vi "Teleop.vi"(10 "Match Info":T1={"Autonomous Elapsed Seconds"=0.0, "TeleOp Elapsed Seconds"=0.0, "Disabled Elapsed Seconds"=0.0, "Visited Autonomous"=FALSE, "Visited TeleOp"=FALSE, "Visited Disabled"=FALSE, "Autonomous Settings"={"Autonomous Style"=enum."Independent", "VI Refnum"=refnum}}, 11 "Call Context":T2) -> ()   [LabVIEW 2011]
doc: "This VI is called for each TeleOp packet received from the DS where the robot is not disabled. It is often used to read from the joysticks and update I/O or to update setpoints for timed control loops. It should complete and return within 20 milliseconds or it may miss DS packets."
uses:
  <vilib>/Rock Robotics/WPI/DriverStation/WPI_DriverStationDerivedRobotMode.ctl
  <vilib>/Rock Robotics/WPI/DriverStation/WPI_DriverStationMatch Info.ctl
  <vilib>/Rock Robotics/WPI/Relay/WPI_RelayValue.ctl
  Robot Global Data.vi
panel:
  out "Shift Control":dbl=2.0 format="%.2f"
  in  "Left High":dbl=0.2
  in  "Right High":dbl=0.8
  in  "Left Mid":dbl=0.25
  in  "Right Mid":dbl=0.7
  in  "Shift Input 2":dbl
  in  "Left Low":dbl=0.8
  in  "Right Low":dbl=0.4
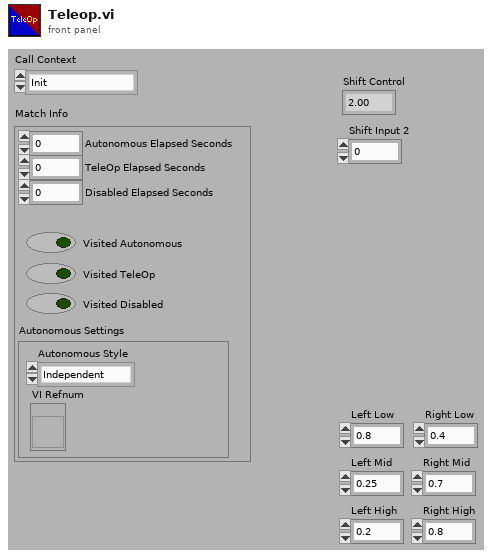
[diagram p1: front panel]
types:
  T1 = typedef "WPI_DriverStationMatch Info.ctl" = cluster{"Autonomous Elapsed Seconds":dbl, "TeleOp Elapsed Seconds":dbl, "Disabled Elapsed Seconds":dbl, "Visited Autonomous":bool, "Visited TeleOp":bool, "Visited Disabled":bool, "Autonomous Settings":cluster{"Autonomous Style":enum16{"Iterative", "Independent"}, "VI Refnum":refnum<vi>}}
  T2 = typedef "WPI_DriverStationDerivedRobotMode.ctl" = enum16{"Init", "Execute", "Stop"}
  T3 = typedef "WPI_RelayValue.ctl" = enum16{"Off", "On", "Forward", "Reverse"}
  T4 = typedef "WPI_MotorControlDeviceRef.ctl" = cluster{"DeviceStatus":errorcluster, "Type":enum16{"PWM", "CAN"}, "PWM":cluster{"Digital Module":T5, "PWM Channel":T6, "DeadBand":T7}, "CAN":cluster{"Device Number":u8, "Control Mode":T8, "Semaphore":T9, "Max Vout":dbl}, "Invert":bool, "TransformRef":T10, "InvTransformRef":T10}
  T5 = typedef "FPGA_TypedefDigitalModule.ctl" = enum16{"Digital Module 1", "Digital Module 2"}
  T6 = typedef "FPGA_DIOPWMChannel.ctl" = enum8{"PWM 1", "PWM 2", "PWM 3", "PWM 4", "PWM 5", "PWM 6", "PWM 7", "PWM 8", "PWM 9", "PWM 10", "Invalid"}
  T7 = typedef "WPI_PWMDeadband.ctl" = cluster{"Name":string, "maxPositivePwm":i32, "minPositivePwm":i32, "centerPwm":i32, "maxNegativePwm":i32, "minNegativePwm":i32, "angularRange":u16}
  T8 = typedef "WPI_CANJaguar_ControlMode.ctl" = enum8{"Percent VBus", "Current", "Speed", "Position", "Voltage"}
  T9 = typedef "Semaphore RefNum" = refnum<k1>
  T10 = typedef "WPI_PWMTransform_ConPane.ctl" = refnum<vi>
  T11 = typedef "WPI_RelayDevRef.ctl" = cluster{"DevStatus":errorcluster, "Relay Channel":T12, "Digital Module":T5, "Relay Direction":T13}
  T12 = typedef "FPGA_DIORelayChannel.ctl" = enum8{"Relay 1", "Relay 2", "Relay 3", "Relay 4", "Relay 5", "Relay 6", "Relay 7", "Relay 8", "Invalid"}
  T13 = typedef "WPI_RelayDirection.ctl" = enum16{"Both directions", "Forward only", "Reverse only"}
  T14 = typedef "WPI_ServoDeviceRef.ctl" = cluster{"DeviceStatus":errorcluster, "Digital Module":T5, "PWM Channel":T6, "DeadBand":T7}
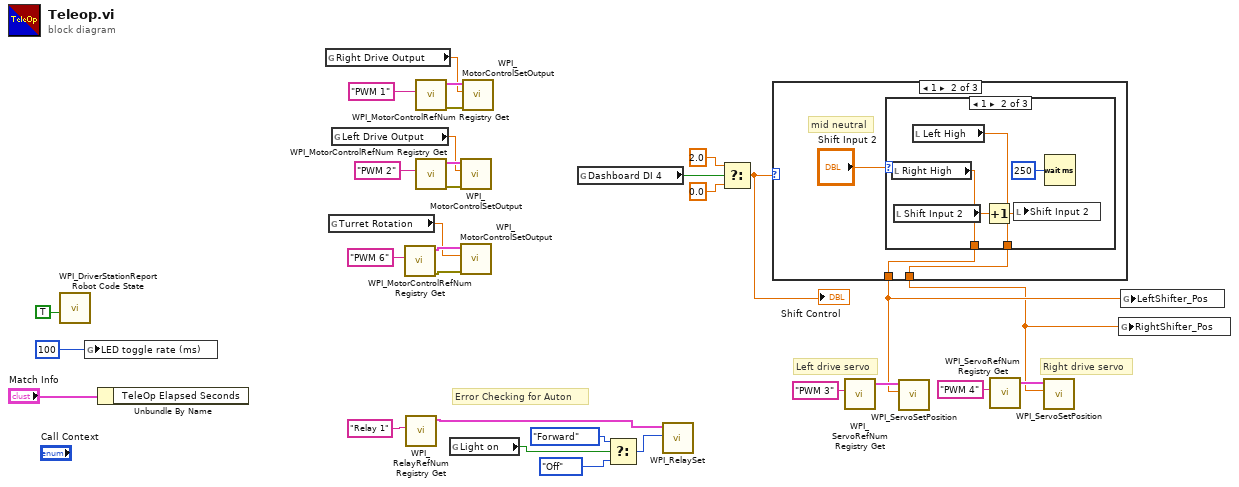
[diagram p0: block diagram]
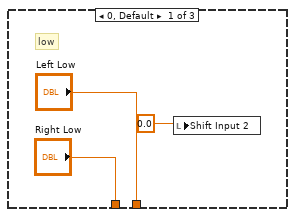
[diagram p2: hidden frame]
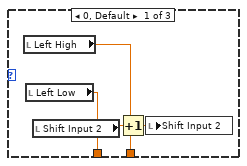
[diagram p3: hidden frame]
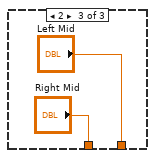
[diagram p4: hidden frame]
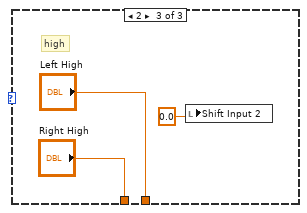
[diagram p5: hidden frame]
diagram:
  # "Error Checking for Auton"
  # "Right drive servo"
  # "Left drive servo"
  n1 = call <vilib>:"WPI_DriverStationReport Robot Code State.vi"("TeleOp"=TRUE ("Autonomous")) -> ()  [unwired: 10 in, 1 out]
  n2 = global write "Robot Global Data.vi" "LED toggle rate (ms)"(u32 100 ("LED ms toggle rate")) -> ()
  n3 = Unbundle By Name("Match Info") -> ()  [unwired: 1 out]
  n4 = global read "Robot Global Data.vi" "Right Drive Output"() -> (w7:dbl)
  n5 = global read "Robot Global Data.vi" "Turret Rotation"() -> (w9:dbl)
  n6 = global read "Robot Global Data.vi" "Left Drive Output"() -> (w8:dbl)
  n7 = call <vilib>:"WPI_MotorControlRefNum Registry Get.vi"("refnum name"="PWM 6") -> ("error out"=w12:errorcluster, "MotorControlDevRef"=w11:T4)  [unwired: 9 in]
  n8 = call <vilib>:"WPI_RelayRefNum Registry Get.vi"("refnum name"="Relay 1") -> ("RelayDevRef"=w1:T11)  [unwired: 9 in, 1 out]
  n9 = call <vilib>:"WPI_MotorControlRefNum Registry Get.vi"("refnum name"="PWM 1") -> ("error out"=w25:errorcluster, "MotorControlDevRef"=w26:T4)  [unwired: 9 in]
  n10 = call <vilib>:"WPI_MotorControlRefNum Registry Get.vi"("refnum name"="PWM 2") -> ("error out"=w23:errorcluster, "MotorControlDevRef"=w24:T4)  [unwired: 9 in]
  n11 = global read "Robot Global Data.vi" "Light on"() -> (w4:bool)
  n12 = call <vilib>:"WPI_MotorControlSetOutput.vi"("error in (no error)"=w23, "Output"=w8, "MotorControlDevRef"=w24) -> ()  [unwired: 7 in, 2 out]
  n13 = call <vilib>:"WPI_MotorControlSetOutput.vi"("error in (no error)"=w12, "Output"=w9, "MotorControlDevRef"=w11) -> ()  [unwired: 7 in, 2 out]
  n14 = call <vilib>:"WPI_MotorControlSetOutput.vi"("error in (no error)"=w25, "Output"=w7, "MotorControlDevRef"=w26) -> ()  [unwired: 7 in, 2 out]
  n15 = global read "Robot Global Data.vi" "Dashboard DI 4"() -> (w15:bool)
  n16 = Select(t=WPI_RelayValue."Forward" ("RelayValue"), s=w4, f=WPI_RelayValue."Off" ("RelayValue")) -> (s? t:f=w3:T3)
  n17 = call <vilib>:"WPI_RelaySet.vi"("RelayValue"=w3, "RelayDevRef"=w1) -> ()  [unwired: 8 in, 2 out]
  n18 = Select(t=2.0, s=w15, f=0.0) -> (s? t:f=w17:dbl)
  "Shift Control" <- w17
  n19 = case shown="1" w17 {
    tunnel: ["Left Low" w36 "Left High"] -> w13
    tunnel: ["Right Low" w35 "Right High"] -> w14
    frame 0, Default {
      # "low"
      n20 = local write "Shift Input 2"(0.0 ("Input 2")) -> ()
    }
    frame 1 {
      # "mid neutral"
      n21 = case shown="1" "Shift Input 2" {
        tunnel: [w41 w42 "Left Mid"] -> w36
        tunnel: [w40 w43 "Right Mid"] -> w35
        frame 0, Default {
          n22 = local read "Left High"() -> (w41:dbl)
          n23 = local read "Left Low"() -> (w40:dbl)
          n24 = local read "Shift Input 2"() -> (w39:dbl)
          n25 = Increment(x=w39) -> (x+1=w38:dbl)
          n26 = local write "Shift Input 2"(w38) -> ()
        }
        frame 1 {
          n27 = local read "Right High"() -> (w43:dbl)
          n28 = local read "Shift Input 2"() -> (w45:dbl)
          n29 = local read "Left High"() -> (w42:dbl)
          n30 = Increment(x=w45) -> (x+1=w44:dbl)
          n31 = local write "Shift Input 2"(w44) -> ()
          n32 = Wait (ms)(milliseconds to wait=u32 250) -> ()  [unwired: 1 out]
        }
        frame 2 {
        }
      }
    }
    frame 2 {
      # "high"
      n33 = local write "Shift Input 2"(0.0 ("Input 2")) -> ()
    }
  }
  n34 = call <vilib>:"WPI_ServoRefNum Registry Get.vi"("refnum name"="PWM 3") -> ("ServoDeviceRef"=w22:T14)  [unwired: 1 in, 9 out]
  n35 = call <vilib>:"WPI_ServoSetPosition.vi"("Position"=w14, "ServoDeviceRef"=w22) -> ()  [unwired: 1 in, 9 out]
  n36 = call <vilib>:"WPI_ServoRefNum Registry Get.vi"("refnum name"="PWM 4") -> ("ServoDeviceRef"=w18:T14)  [unwired: 1 in, 9 out]
  n37 = call <vilib>:"WPI_ServoSetPosition.vi"("Position"=w13, "ServoDeviceRef"=w18) -> ()  [unwired: 1 in, 9 out]
  n38 = global write "Robot Global Data.vi" "RightShifter_Pos"(w13) -> ()
  n39 = global write "Robot Global Data.vi" "LeftShifter_Pos"(w14) -> ()
